vi "INI_PicoScope.vi"(3 "MCListbox Ref":refnum<vi>, 8 "MListBox Row":u16=2 max=8, 10 "Device INI Config File Path":path=path "D:/LABVIEW/SEQUENSER SNA/Ver 07/INI") -> (0 "error out":errorcluster, 1 "Handle":u32, 2 "Dev OK":bool, 4 "Device Info":T1, 5 "Max Adc value":i16, 6 "PicoScope Correction":i32)   [LabVIEW 2018]
uses:
  <vilib>/Utility/miscctls.llb/LVRowAndColumnTypeDef.ctl
  <vilib>/Utility/config.llb/Read Key (String).vi
  <vilib>/Utility/config.llb/Read Key (I32).vi
  <vilib>/Utility/config.llb/NI_LVConfig.lvlib
panel:
  out "Serial Number":string
  out "PicoScope Type":string
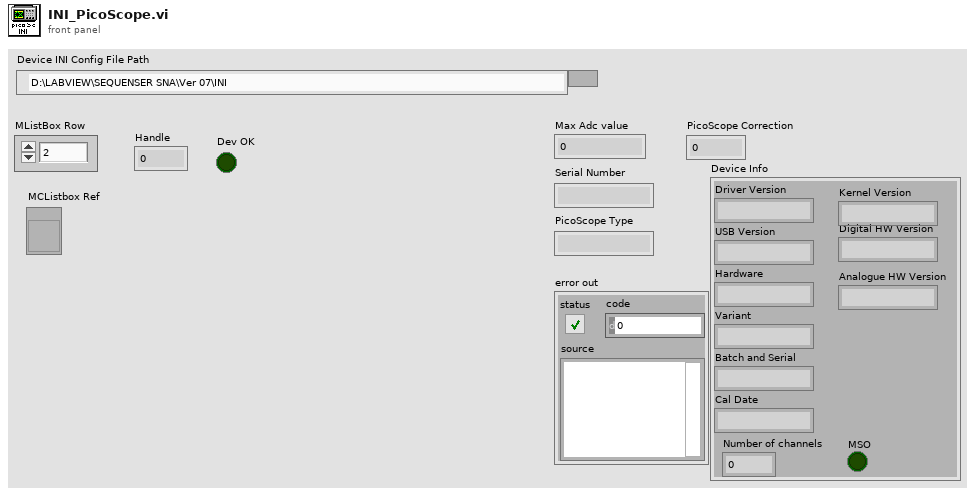
[diagram p1: front panel]
types:
  T1 = cluster{"Driver Version":string, "USB Version":string, "Hardware":string, "Variant":string, "Batch and Serial":string, "Cal Date":string, "Kernel Version":string, "Digital HW Version":string, "Analogue HW Version":string, "MSO":bool, "Number of channels":i16}
  T2 = typedef "LVRowAndColumnTypeDef.ctl" = cluster{"Row":i32, "Column":i32}
  T3 = typedef "NI_LVConfig.lvlib/Config Data RefNum.ctl" = refnum<k1>
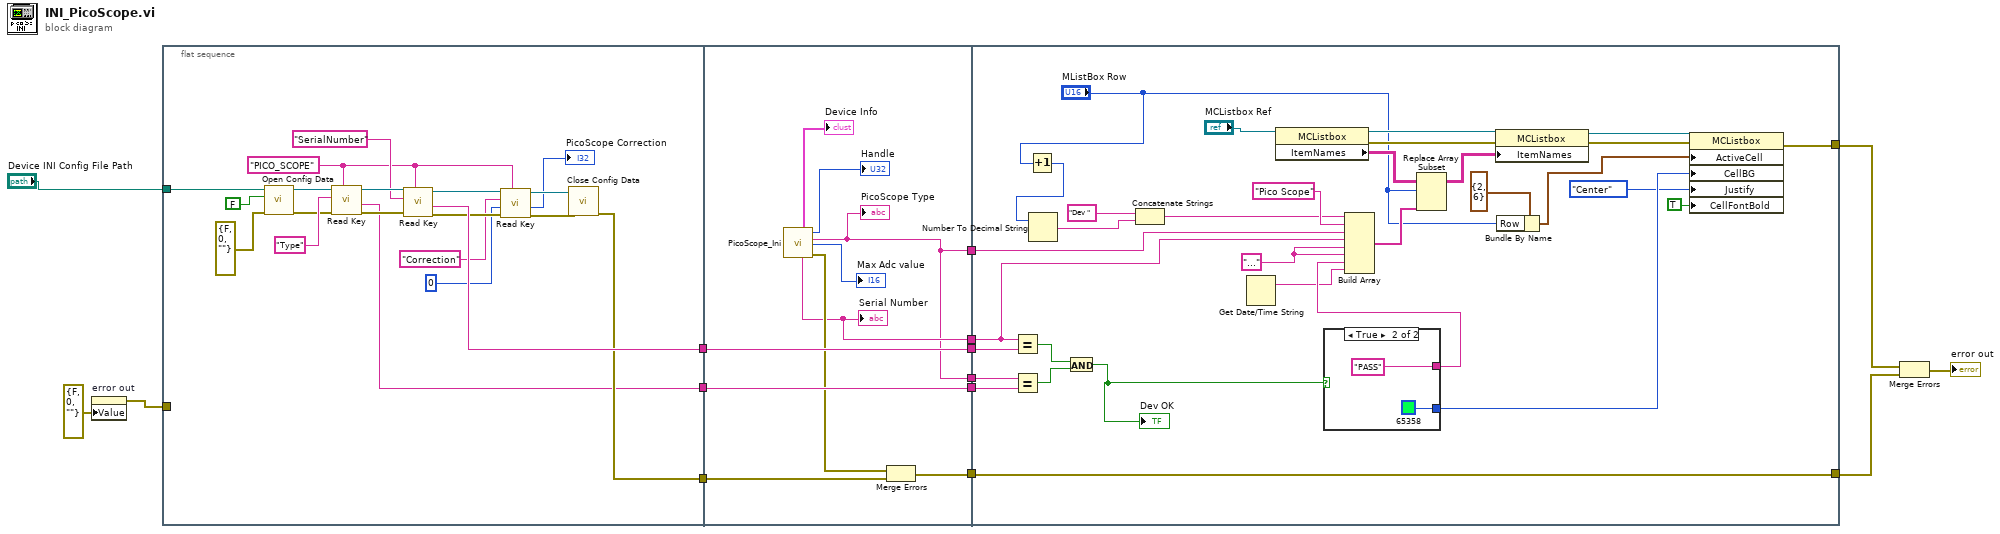
[diagram p0: block diagram]
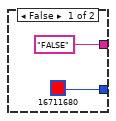
[diagram p2: hidden frame]
diagram:
  n1 = property on="error out" class="Clust (strict)"("Value"=errorcluster {"status"=FALSE, "code"=0, "source"=""} ("error out")) -> (error out=w4:errorcluster)  [unwired: 2 in, 1 out]
  n2 = flat-sequence {
    tunnel: "Device INI Config File Path" -> [w30]
    tunnel: [w26] -> w15
    tunnel: [w25] -> w14
    tunnel: [w24] -> w10
    tunnel: w4 -> [_]
    tunnel: w15 -> [w42]
    tunnel: w14 -> [w43]
    tunnel: [w45] -> w11
    tunnel: w10 -> [w45]
    tunnel: [w44] -> w9
    tunnel: [w42] -> w8
    tunnel: [w39] -> w7
    tunnel: [w38] -> w6
    tunnel: [w38] -> w5
    tunnel: [w57] -> w2
    tunnel: [w56] -> w1
    tunnel: w11 -> [w55]
    tunnel: w9 -> [w56]
    tunnel: w8 -> [w51]
    tunnel: w7 -> [w46]
    tunnel: w6 -> [w47]
    tunnel: w5 -> [w52]
    frame #0 {
      w19 = "PICO_SCOPE" ("section")
      n3 = call <vilib>:"Open Config Data.vi"("error in (no error)"=errorcluster {"status"=FALSE, "code"=0, "source"=""} ("error constant"), "create file if necessary (T)"=FALSE, "configuration file path"=w30) -> ("error out"=w33:errorcluster, "refnum"=w32:T3)  [unwired: 6 in, 1 out]
      n4 = call-poly <vilib>:"Read Key.vi"("section"=w19, "error in (no error)"=w33, "key"="Type", "refnum"=w32) -> ("error out"=w28:errorcluster, "value"=w24:string, "refnum out"=w29:T3)  [unwired: 4 in, 1 out]
      n5 = call-poly <vilib>:"Read Key.vi"("section"=w19, "error in (no error)"=w28, "key"="SerialNumber", "refnum"=w29) -> ("error out"=w23:errorcluster, "value"=w26:string, "refnum out"=w21:T3)  [unwired: 4 in, 1 out]
      n6 = call-poly <vilib>:"Read Key.vi"("section"=w19, "error in (no error)"=w23, "default value"=0, "key"="Correction", "refnum"=w21) -> ("error out"=w22:errorcluster, "value"=→"PicoScope Correction":i32, "refnum out"=w20:T3)  [unwired: 3 in, 1 out]
      n7 = call <vilib>:"Close Config Data.vi"("error in (no error)"=w22, "refnum"=w20) -> ("error out"=w25:errorcluster)  [unwired: 8 in, 1 out]
    }
    frame #1 {
      n8 = call "PicoScope_Ini.vi"() -> ("error out"=w41:errorcluster, "Max Adc value"=→"Max Adc value":i16, "PicoScope Type"=w38:string, "handle"=→"Handle":i16, "Serial"=w39:string, "Device Info"=→"Device Info":T1)  [unwired: 6 in]
      "PicoScope Type" <- w38
      "Serial Number" <- w39
      n9 = Merge Errors(w41, w43) -> (w44:errorcluster)
    }
    frame #2 {
      w77 = "..."
      n10 = Equal?(x=w46, y=w51) -> (x = y?=w50:bool)
      n11 = Equal?(x=w52, y=w55) -> (x = y?=w49:bool)
      n12 = Increment(x="MListBox Row") -> (x+1=w54:u16)
      n13 = Number To Decimal String(number=w54) -> (decimal integer string=w74:string)  [unwired: 1 in]
      n14 = And(x=w50, y=w49) -> (x .and. y?=w48:bool)
      "Dev OK" <- w48
      n15 = Concatenate Strings("Dev ", w74) -> (w75:string)
      n16 = Get Date/Time String() -> (date string=w67:string)  [unwired: 3 in, 1 out]
      n17 = property class="MCListbox"(reference="MCListbox Ref") -> (reference out=w65:refnum<vi>, error out=w64:errorcluster, "ItemNames"=w63:string[][])  [unwired: 1 in]
      n18 = case shown="True" w48 {
        tunnel: [u32 16711680 u32 65358] -> w70
        tunnel: ["FALSE" ("element") "PASS" ("element")] -> w71
        frame False {
        }
        frame True {
        }
      }
      n19 = Build Array(w75, "Pico Scope", w47, w46, w77, w77, w71, w67) -> (w61:string[])
      n20 = Replace Array Subset(array=w63, new element=w61, index (row)="MListBox Row") -> (w62:string[][])  [unwired: 1 in]
      n21 = property class="MCListbox"(reference=w65, error in=w64, "ItemNames"=w62) -> (reference out=w60:refnum<vi>, error out=w59:errorcluster)
      n22 = Bundle By Name(cluster=T2 {"Row"=2, "Column"=6} ("Active Cell:Active Cell"), "Row"="MListBox Row") -> (w69:T2)
      n23 = property class="MCListbox"(reference=w60, error in=w59, "ActiveCell"=w69, "CellBG"=w70, "Justify"=enum16{"Left", "Center", "Right"}."Center" ("Active Cell:Cell Justification"), "CellFontBold"=TRUE ("Active Cell:Cell Font:Bold")) -> (error out=w57:errorcluster)  [unwired: 1 out]
    }
  }
  n24 = Merge Errors(w2, w1) -> (→"error out":errorcluster)
